vi "_OBSOLETE_PathPlanner_Trajectory_GeneratePath.vi"(8 "Reversed":bool, 9 "MaxAccel":dbl, 10 "MaxVel":dbl, 11 "PathPoints":T5[](array[typedef]) {"HolonomicRotation"."SIN" format="%13.4f"; "HolonomicRotation"."COS" format="%13.4f"; "HolonomicRotation"."VALUE" format="%13.4f"; "NextControl"."Y" format="%14.3f"; "NextControl"."X" format="%14.3f"; "PrevControl"."Y" format="%14.3f"; "PrevControl"."X" format="%14.3f"; "AnchorPoint"."Y" format="%14.3f"; "AnchorPoint"."X" format="%14.3f"}) -> (3 "PathPlannerStates":T1[](array[typedef]) {"TargetHolonomicRotation"."SIN" format="%13.4f"; "TargetHolonomicRotation"."COS" format="%13.4f"; "TargetHolonomicRotation"."VALUE" format="%13.4f"; "Heading"."SIN" format="%13.4f"; "Heading"."COS" format="%13.4f"; "Heading"."VALUE" format="%13.4f"; "PositionMeters"."Y" format="%14.3f"; "PositionMeters"."X" format="%14.3f"})   [LabVIEW 2019]
uses:
  PathPlanner24.lvlib
  <vilib>/Rock Robotics/WPI/ThirdParty/JAS_Junk/TrajLib/TypeDef/TRANSLATION2D.ctl
  <vilib>/Rock Robotics/WPI/ThirdParty/JAS_Junk/TrajLib/Trajectory_Library.lvlib
  <vilib>/Rock Robotics/WPI/ThirdParty/JAS_Junk/TrajLib/TypeDef/ROTATION2D.ctl
  TypeDef/PathPlannerWaypoint.ctl
  TypeDef/PathPlannerTrajectoryState.ctl
  TypeDef/PathPlannerPathConstraints.ctl
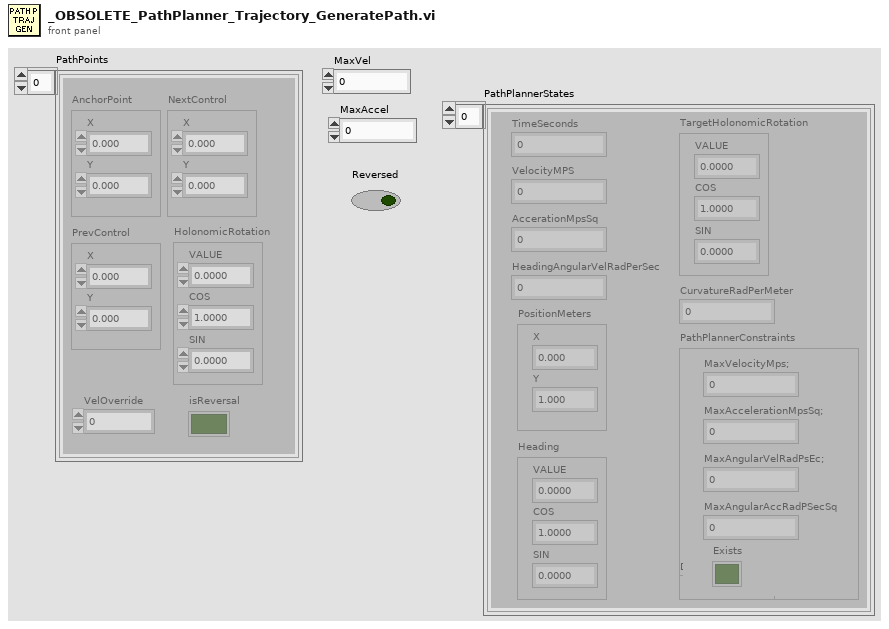
[diagram p1: front panel]
types:
  T1 = typedef "PathPlanner24.lvlib/PathPlannerTrajectoryState.ctl" = cluster{"TimeSeconds":dbl, "VelocityMPS":dbl, "AccerationMpsSq":dbl, "HeadingAngularVelRadPerSec":dbl, "PositionMeters":T2, "Heading":T3, "TargetHolonomicRotation":T3, "CurvatureRadPerMeter":dbl, "DeltaPos":dbl, "PathPlannerConstraints":T4}
  T2 = typedef "Trajectory_Library.lvlib/TRANSLATION2D.ctl" = cluster{"X":dbl, "Y":dbl}
  T3 = typedef "Trajectory_Library.lvlib/ROTATION2D.ctl" = cluster{"VALUE":dbl, "COS":dbl, "SIN":dbl}
  T4 = typedef "PathPlanner24.lvlib/PathPlannerPathConstraints.ctl" = cluster{"MaxVelocityMps;":dbl, "MaxAccelerationMpsSq;":dbl, "MaxAngularVelRadPsEc;":dbl, "MaxAngularAccRadPSecSq":dbl, "Exists":bool}
  T5 = typedef "PathPlanner24.lvlib/PathPlannerWaypoint.ctl" = cluster{"AnchorPoint":T2, "PrevControl":T2, "NextControl":T2, "HolonomicRotation":T3, "VelOverride":dbl, "isReversal":bool}
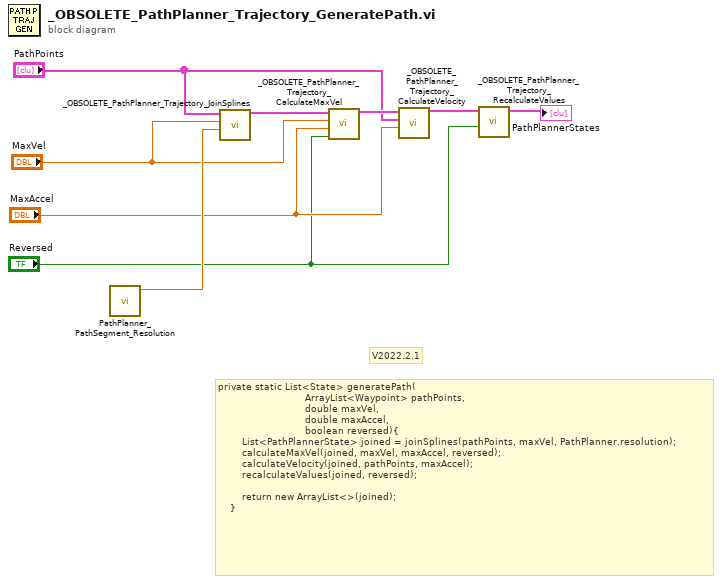
[diagram p0: block diagram]
diagram:
  # "private static List<State> generatePath(\n                             ArrayList<Waypoint> pathPoints, \n                             double maxVel, \n                             double maxAccel, \n                             boolean reversed){\n        List<PathPlannerState> joined = joinSplines(pathPoints, maxVel, PathPlanner.resolution);\n        calculateMaxVel(joined, maxVel, maxAccel, reversed);\n        calculateVelocity(joined, pathPoints, maxAccel);\n        recalculateValues(joined, reversed);\n\n        return new ArrayList<>(joined);\n    }"
  # "V2022.2.1"
  n1 = call "PathPlanner_PathSegment_Resolution.vi"() -> ("Resolution"=w9:dbl)  [unwired: 11 in]
  n2 = call "_OBSOLETE_PathPlanner_Trajectory_JoinSplines.vi"("Step"=w9, "Max Velocity"="MaxVel", "PathPoints"="PathPoints") -> ("outPathPlannerStates"=w8:T1[])  [unwired: 8 in]
  n3 = call "_OBSOLETE_PathPlanner_Trajectory_CalculateMaxVel.vi"("Reversed"="Reversed", "MaxAccel"="MaxAccel", "MaxVel"="MaxVel", "PathPlannerStates"=w8) -> ("outPathPlannerStates"=w6:T1[])  [unwired: 7 in]
  n4 = call "_OBSOLETE_PathPlanner_Trajectory_CalculateVelocity.vi"("MaxAccel"="MaxAccel", "PathPoints"="PathPoints", "PathPlannerStates"=w6) -> ("outPathPlannerStates"=w3:T1[])  [unwired: 8 in]
  n5 = call "_OBSOLETE_PathPlanner_Trajectory_RecalculateValues.vi"("Reversed"="Reversed", "PathPlannerStates"=w3) -> ("outPathPlannerStates"=→"PathPlannerStates":T1[])  [unwired: 9 in]
